vi "Start.vi"(8 "error in (no error)":errorcluster, 11 "TCPMessaging in":refnum<class "TCPMessaging.lvclass">) -> (0 "error out":errorcluster, 3 "TCPMessaging out":refnum<class "TCPMessaging.lvclass">)   [LabVIEW 2020, in "Vecto.lvlib" / "TCPMessaging.lvclass"]
uses:
  TCPMessaging.lvclass
  TCPMessaging.lvclass/TCPMessaging.ctl
  Client Loops.vi
  Server Loops.vi
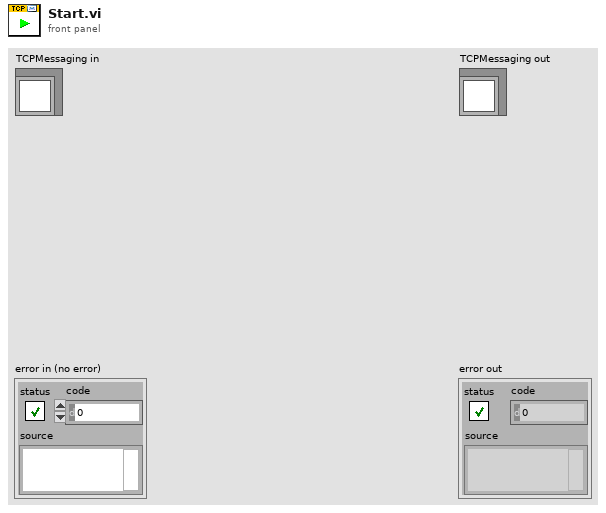
[diagram p1: front panel]
types:
  T1 = typedef "Vecto.lvlib/TCPMessaging.lvclass/TCP Mode.ctl" = enum16{"Client", "Server"}
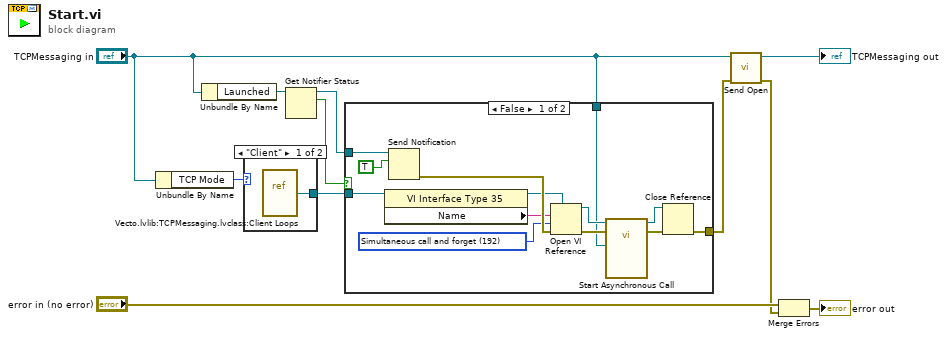
[diagram p0: block diagram]
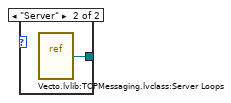
[diagram p3: hidden frame]
diagram:
  n1 = Unbundle By Name("TCPMessaging in") -> ("TCP Mode"=w10:T1)
  n2 = Unbundle By Name("TCPMessaging in") -> ("Launched"=w7:refnum<notifier>)
  n3 = case shown="\"Client\"" w10 {
    tunnel: [w12 w13] -> w8
    frame "Client" {
      n4 = vi-ref "Vecto.lvlib:TCPMessaging.lvclass:Client Loops.vi"() -> (w12:refnum<vi>)
    }
    frame "Server" {
      n5 = vi-ref "Vecto.lvlib:TCPMessaging.lvclass:Server Loops.vi"() -> (w13:refnum<vi>)
    }
  }
  n6 = Get Notifier Status(notifier=w7) -> (notifier out=w5:refnum<notifier>, current notification=w6:bool)  [unwired: 1 in, 3 out]
  n7 = case shown="False" w6 {
    tunnel: w8 -> [w18 _]
    tunnel: w5 -> [w17 _]
    tunnel: [w15 _] -> w2
    tunnel: "TCPMessaging in" -> [w14 _]
    frame False {
      w19 = 192 items=["Record modifications"=1, "Open templates for editing"=2, "Prompt user to save"=4, "Prepare for reentrant run"=8, "Prompt to find missing subVIs"=16, "Hide loading dialog box"=32, "Enable simultaneous calls"=64, "Prepare to call and forget"=128, "Simultaneous call and forget"=192, "Prepare to call and collect"=256, "Simultaneous call and collect"=320]
      n8 = property class="VI Interface Type 35"(reference=w18) -> (reference out=w21:refnum<vi>, "Name"=w20:string)  [unwired: 1 in, 1 out]
      n9 = Send Notification(notification=TRUE, notifier=w17) -> (error out=w26:errorcluster)  [unwired: 1 in, 1 out]
      n10 = Open VI Reference(type specifier VI Refnum (for type only)=w21, vi path=w20, options=w19, error in (no error)=w26) -> (vi reference=w23:refnum<vi>, error out=w22:errorcluster)  [unwired: 2 in]
      n11 = call-by-ref "Start Asynchronous Call"(reference=w23, error in=w22, "TCPMessaging in"=w14) -> (reference out=w25:refnum<vi>, error out=w24:errorcluster)  [unwired: 11 in]
      n12 = Close Reference(reference=w25, error in (no error)=w24) -> (error out=w15:errorcluster)
    }
    frame True {
    }
  }
  n13 = call "Send Open.vi"("error in (no error)"=w2, "TCPMessaging in"="TCPMessaging in") -> ("error out"=w1:errorcluster, "TCPMessaging out"=→"TCPMessaging out":refnum<class "TCPMessaging.lvclass">)  [unwired: 8 in]
  n14 = Merge Errors("error in (no error)", w1) -> (→"error out":errorcluster)
